vi "Set image label attributes.vi"(7 "Enable dynamic stream change?":bool, 8 "error in (no error)":errorcluster, 9 "Rack deatils":cluster{"ISIM":u8[], "#Racks":i32}, 10 "Dynamic image update params":T1, 11 "Label array":refnum<vi>[](array[refnum])) -> (0 "error out":errorcluster)   [LabVIEW 2019, in "ZenGage v3.0 UI.lvclass"]
uses:
  ZenGage v3.0 UI.lvclass
panel:
  out "Mapped view names":string[](array[string])
  in  "Camera Names":string[](array[string])
  in  "CameraLabelMapping":T2(array[cluster])
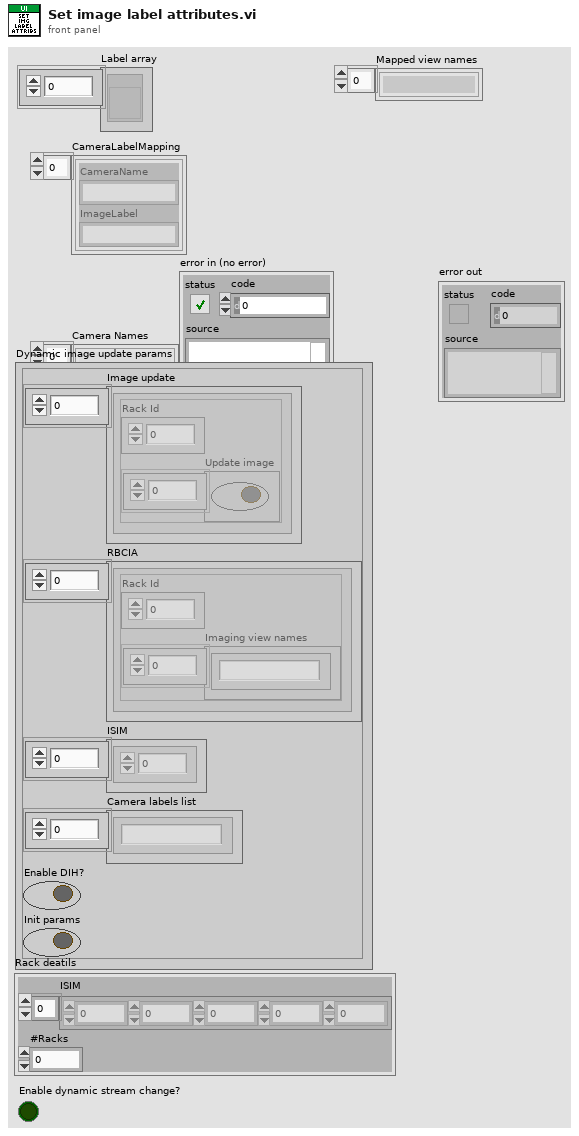
[diagram p1: front panel]
types:
  T1 = cluster{"Image update":cluster{"Rack Id":i32, "Update image":bool[]}[], "RBCIA":cluster{"Rack Id":u8, "Imaging view names":string[]}[], "ISIM":u8[], "Camera labels list":string[], "Enable DIH?":bool, "Init params":bool}
  T2 = cluster{"CameraName":string, "ImageLabel":string}[]
  T3 = enum8{"Enabled", "Disabled", "Disabled and Grayed Out"}
  T4 = cluster{"Rack Id":u8, "Imaging view names":string[]}[]
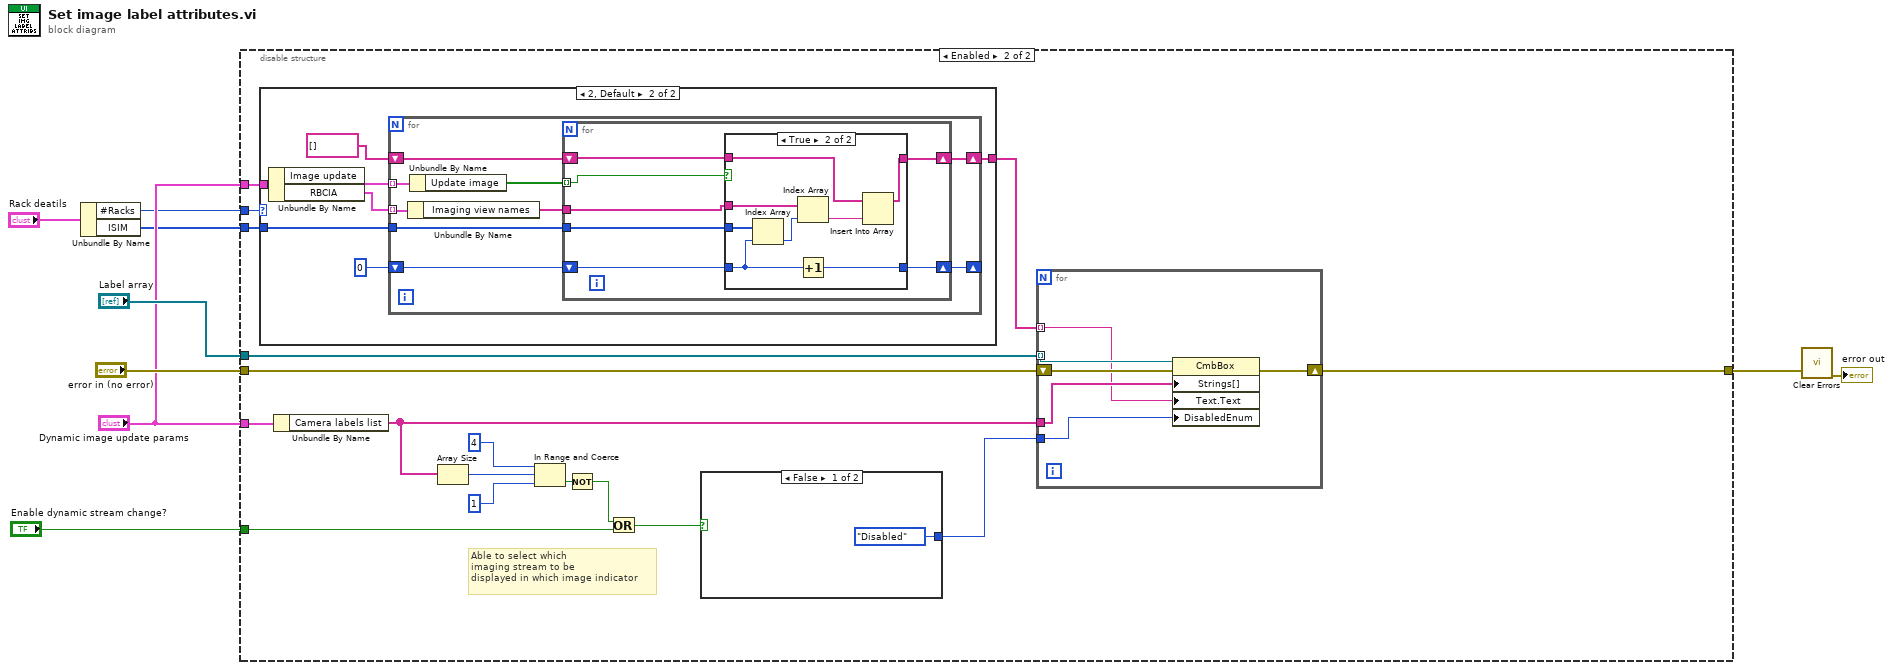
[diagram p0: block diagram]
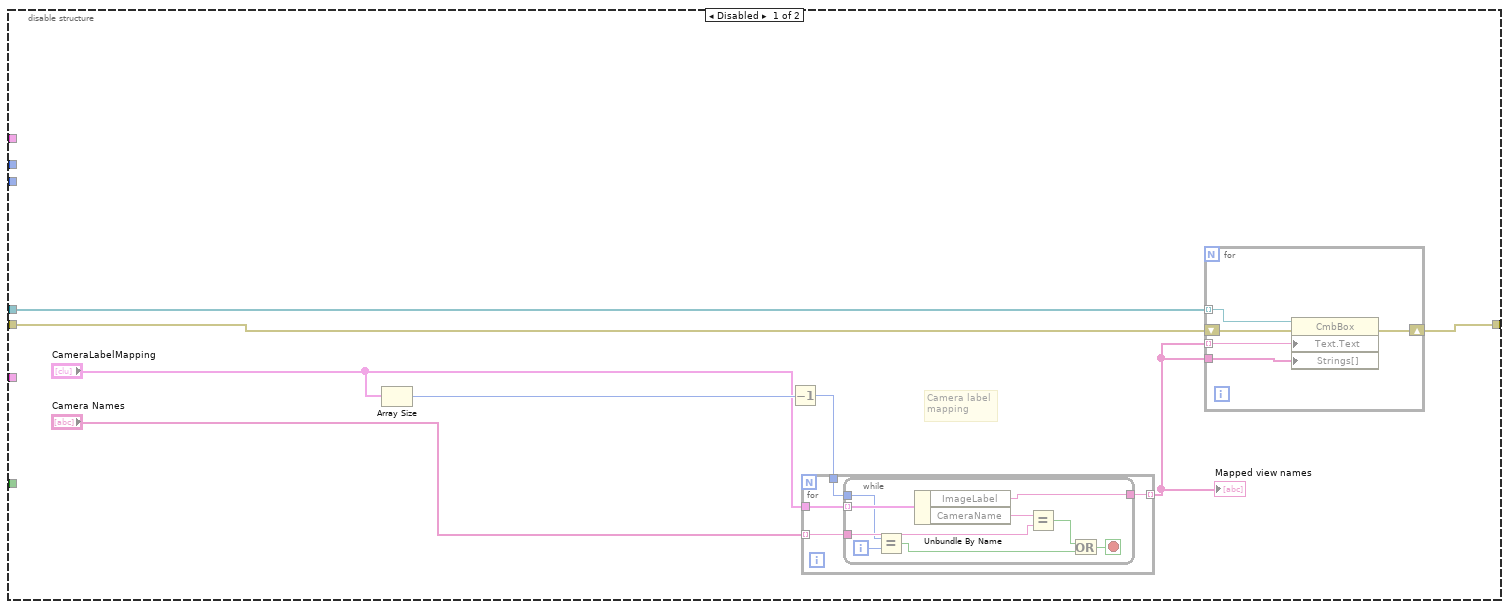
[diagram p2: hidden frame]
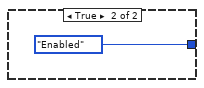
[diagram p3: hidden frame]
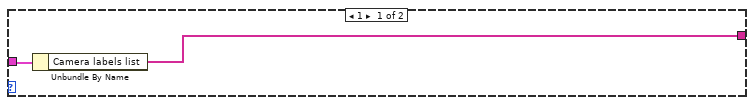
[diagram p4: hidden frame]
diagram:
  n1 = Unbundle By Name("Rack deatils") -> ("#Racks"=w2:i32, "ISIM"=w3:u8[])
  n2 = disable-structure shown="Enabled" {
    disable-tunnel: "error in (no error)" -> [w14 w50]
    disable-tunnel: "Label array" -> [w13 w52]
    disable-tunnel: [w12 w49] -> w7
    disable-tunnel: "Dynamic image update params" -> [_ w51]
    disable-tunnel: "Dynamic image update params" -> [_ w48]
    disable-tunnel: w3 -> [_ w47]
    disable-tunnel: w2 -> [_ w45]
    disable-tunnel: "Enable dynamic stream change?" -> [_ w37]
    frame Disabled {
      # "Camera label\nmapping"
      n3 = Array Size(array="CameraLabelMapping") -> (size(s)=w16:i32)
      n4 = Decrement(x=w16) -> (x-1=w17:i32)
      n5 = for {
        tunnel: "CameraLabelMapping" -> [w24]
        tunnel: "Camera Names" -> [w26] mode=indexing
        tunnel: [w25] -> w10 mode=indexing
        tunnel: w17 -> [w23]
        n6 = while {
          tunnel: w26 -> [w35]
          tunnel: w24 -> [w34] mode=indexing
          tunnel: [w32] -> w25
          tunnel: w23 -> [w30]
          i -> [w31]
          stop <- w29 stop-if-true
          n7 = Equal?(x=w30, y=w31) -> (x = y?=w27:bool)
          n8 = Unbundle By Name(w34) -> ("ImageLabel"=w32:string, "CameraName"=w33:string)
          n9 = Equal?(x=w33, y=w35) -> (x = y?=w28:bool)
          n10 = Or(x=w28, y=w27) -> (x .or. y?=w29:bool)
        }
      }
      "Mapped view names" <- w10
      n11 = for {
        tunnel: w13 -> [w21] mode=indexing
        tunnel: w10 -> [w20] mode=indexing
        shift-right: [w19] -> w12
        shift-left: w14 -> [w22]
        tunnel: w10 -> [w18]
        n12 = property class="CmbBox"(reference=w21, error in=w22, "Text.Text"=w20, "Strings[]"=w18) -> (error out=w19:errorcluster)  [unwired: 1 out]
      }
    }
    frame Enabled {
      # "Able to select which\nimaging stream to be\ndisplayed in which image indicator"
      n13 = case shown="2, Default" w45 {
        tunnel: w48 -> [w56 w63]
        tunnel: w47 -> [_ w58]
        tunnel: [w55 w57] -> w46
        frame 1 {
          n14 = Unbundle By Name(w56) -> ("Camera labels list"=w55:string[])
        }
        frame 2, Default {
          n15 = Unbundle By Name(w63) -> ("Image update"=w62:cluster{"Rack Id":i32, "Update image":bool[]}[], "RBCIA"=w61:T4)
          n16 = for {
            tunnel: w62 -> [w72] mode=indexing
            tunnel: w61 -> [w65] mode=indexing
            shift-right: [w69] -> _
            shift-left: 0 -> [w70]
            shift-right: [w67] -> w57
            shift-left: string[] [] ("array") -> [w68]
            tunnel: w58 -> [w66]
            n17 = Unbundle By Name(w65) -> ("Imaging view names"=w64:string[])
            n18 = Unbundle By Name(w72) -> ("Update image"=w71:bool[])
            n19 = for {
              tunnel: w71 -> [w79] mode=indexing
              shift-right: [w77] -> w69
              shift-left: w70 -> [w78]
              shift-right: [w75] -> w67
              shift-left: w68 -> [w76]
              tunnel: w66 -> [w74]
              tunnel: w64 -> [w73]
              n20 = case shown="True" w79 {
                tunnel: w73 -> [_ w89]
                tunnel: w78 -> [w81 w83]
                tunnel: [w81 w88] -> w77
                tunnel: w76 -> [w80 w86]
                tunnel: [w80 w85] -> w75
                tunnel: w74 -> [_ w84]
                frame False {
                }
                frame True {
                  n21 = Index Array(array=w84, index=w83) -> (element=w82:u8)
                  n22 = Index Array(array=w89, index=w82) -> (element=w87:string)
                  n23 = Increment(x=w83) -> (x+1=w88:i32)
                  n24 = Insert Into Array(array=w86, new element=w87) -> (w85:string[])  [unwired: 1 in]
                }
              }
            }
          }
        }
      }
      n25 = Unbundle By Name(w51) -> ("Camera labels list"=w43:string[])
      n26 = Array Size(array=w43) -> (size(s)=w42:i32)
      n27 = In Range and Coerce(upper limit=4, x=w42, lower limit=1) -> (In Range?=w39:bool)  [unwired: 1 out]
      n28 = Not(x=w39) -> (.not. x?=w38:bool)
      n29 = Or(x=w38, y=w37) -> (x .or. y?=w36:bool)
      n30 = case shown="False" w36 {
        tunnel: [T3."Disabled" ("Disabled") T3."Enabled" ("Disabled")] -> w44
        frame False {
        }
        frame True {
        }
      }
      n31 = for {
        tunnel: w52 -> [w95] mode=indexing
        tunnel: w43 -> [w94]
        shift-right: [w92] -> w49
        shift-left: w50 -> [w93]
        tunnel: w46 -> [w91] mode=indexing
        tunnel: w44 -> [w90]
        n32 = property class="CmbBox"(reference=w95, error in=w93, "Strings[]"=w94, "Text.Text"=w91, "DisabledEnum"=w90) -> (error out=w92:errorcluster)  [unwired: 1 out]
      }
    }
  }
  n33 = call <vilib>:"Clear Errors.vi"("error in (no error)"=w7) -> ("error out"=→"error out":errorcluster)  [unwired: 5 in, 1 out]
